vi "FTW-Actor-InitializeTagEngine.vi"(0 "FTW Actor Instance Type":refnum<class "FTW-ActorInstance.lvclass">, 7 "Actor Instance Configuration":string, 11 "error in":errorcluster) -> (4 "FTW Actor Instance":refnum<class "FTW-ActorInstance.lvclass">, 15 "error out":errorcluster)   [LabVIEW 2018, in "FTW-ActorInstance.lvclass"]
uses:
  FTW-ActorInstance.lvclass
  FTW-ActorInstance.lvclass/FTW-ActorInstance.ctl
  77ebd7b1-2cdb-4688-b895-e9a2b230ff2d.vi
  JSON/core/FTW-JSON-Core-EncodingFlags.vi
  Reflection/FTW-Reflection-Type.vi
  JSON/FTW-JSON-Parse.vi
  container/FTW-Container-GetFlattenedValue.vi
  Ether/FTW-Ether.lvclass
panel:
  # "Inputs"
  # "Outputs"
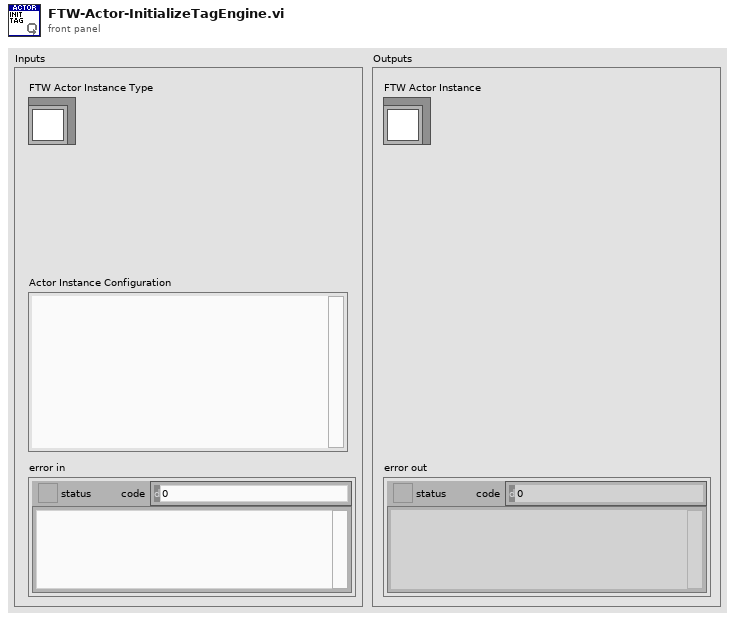
[diagram p1: front panel]
types:
  T1 = cluster{string, "TagAddress":string, "Tag Connection":refnum<class "FTW-ActorConnector.lvclass">, bool}
  T2 = cluster{"Name":string, "URI":string, "Connector":refnum<class "FTW-ActorConnector.lvclass">, "Child":bool}[]
  T3 = cluster{"Name":string, "TagAddress":string, "Tag Connection":refnum<class "FTW-ActorConnector.lvclass">, "Child":bool}[]
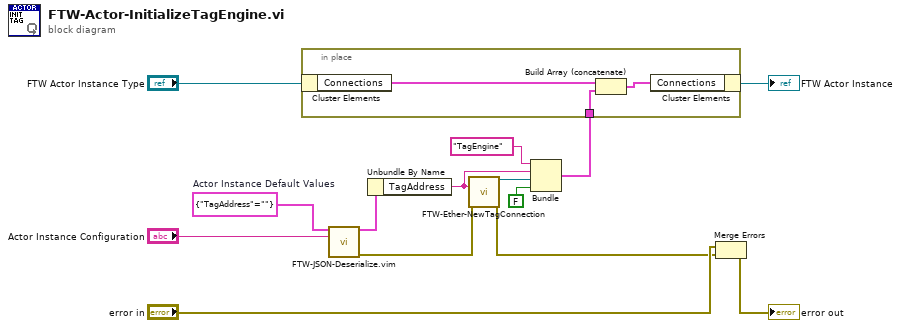
[diagram p0: block diagram]
diagram:
  w8 = cluster{"TagAddress":string} {"TagAddress"=""}  # Actor Instance Default Values
  n1 = call "FTW-JSON-Deserialize.vim"("Type In"=w8, "JSON String"="Actor Instance Configuration") -> ("Type Out"=w13:cluster{"TagAddress":string}, "error out"=w12:errorcluster)  [unwired: 12 in]
  n2 = Unbundle By Name(w13) -> ("TagAddress"=w2:string)
  n3 = call "FTW-Ether-NewTagConnection.vi"("Tag Address"=w2, "error in"=w12) -> ("Tag Connection"=w4:refnum<class "FTW-ActorConnector.lvclass">, "error out"=w9:errorcluster)  [unwired: 12 in]
  n4 = Bundle("TagEngine", "TagAddress"=w2, "Tag Connection"=w4, FALSE) -> (w5:T1)  [unwired: 1 in]
  n5 = in-place {
    in-place-border: w5 -> [w15]
    n6 = in-place-cluster #1("FTW Actor Instance Type") -> ("Connections"=w17:T2)
    n7 = Build Array (concatenate)(w17, w15) -> (w16:T3)
    n8 = in-place-cluster #1("Connections"=w16) -> (→"FTW Actor Instance":refnum<class "FTW-ActorInstance.lvclass">)
  }
  n9 = Merge Errors("error in", w9) -> (→"error out":errorcluster)
